vi "combine time and data into a single array.vi"() -> ()   [LabVIEW 2011]
uses:
  <vilib>/Utility/file.llb/Write To Spreadsheet File (DBL).vi
panel:
  in  "name of file":string="test data.txt"
  in  "export path 2":path=path "C:/Users/VGroup/Desktop/testing file"
  in  "seconds to wait":u32=1
  in  "stop":bool
  out "appended array":dbl[](array[numeric])=[51.0, 140621.0, 200625.0, 0.14448535757155878]
  out "date number":i32=140621
  out "time number":i32=200625
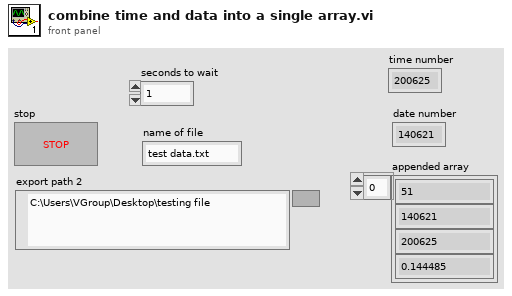
[diagram p1: front panel]
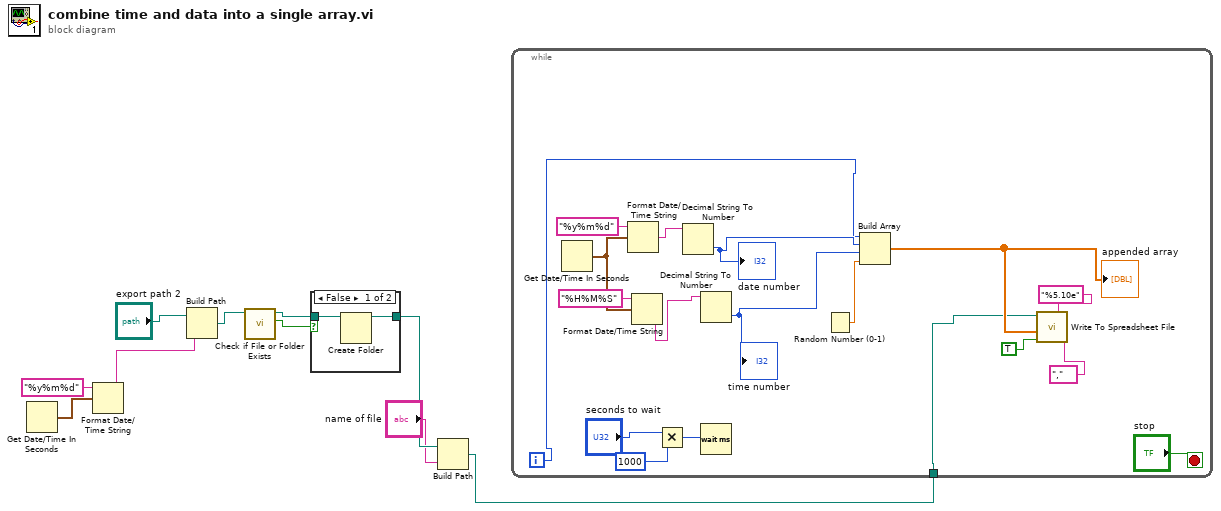
[diagram p0: block diagram]
diagram:
  n1 = Get Date/Time In Seconds() -> (seconds since 1Jan1904=w6:timestamp)
  n2 = Format Date/Time String(time format string (%c)="%y%m%d", seconds (now)=w6) -> (date/time string=w5:string)  [unwired: 1 in]
  n3 = Build Path(base path="export path 2", name or relative path=w5) -> (appended path=w3:path)
  n4 = call <vilib>:"Check if File or Folder Exists.vi"("path"=w3) -> ("file or folder exists?"=w1:bool, "dup path"=w2:path)  [unwired: 8 in, 1 out]
  n5 = case shown="False" w1 {
    tunnel: [w12 w13] -> w9
    tunnel: w2 -> [w11 w13]
    frame False {
      n6 = Create Folder(path (use dialog)=w11) -> (created path=w12:path)  [unwired: 2 in, 2 out]
    }
    frame True {
    }
  }
  n7 = Build Path(base path=w9, name or relative path="name of file") -> (appended path=w7:path)
  n8 = while {
    tunnel: w7 -> [w17]
    i -> [w21]
    stop <- "stop" stop-if-true
    n9 = Get Date/Time In Seconds() -> (seconds since 1Jan1904=w31:timestamp)
    n10 = Format Date/Time String(time format string (%c)="%y%m%d", seconds (now)=w31) -> (date/time string=w14:string)  [unwired: 1 in]
    n11 = Format Date/Time String(time format string (%c)="%H%M%S", seconds (now)=w31) -> (date/time string=w30:string)  [unwired: 1 in]
    n12 = Multiply(x="seconds to wait", y=u32 1000) -> (x*y=w18:u32)
    n13 = Decimal String To Number(string=w14) -> (number=w28:i32)  [unwired: 2 in, 1 out]
    "date number" <- w28
    n14 = Decimal String To Number(string=w30) -> (number=w27:i32)  [unwired: 2 in, 1 out]
    "time number" <- w27
    n15 = Wait (ms)(milliseconds to wait=w18) -> ()  [unwired: 1 out]
    n16 = Random Number (0-1)() -> (number: 0 to 1=w29:dbl)
    n17 = Build Array(w21, w28, w27, w29) -> (w24:dbl[])
    "appended array" <- w24
    n18 = call-poly <vilib>:"Write To Spreadsheet File.vi"("delimiter (\\t)"="," ("delimiter (Tab)"), "format (%.3f)"="%5.10e", "append to file? (new file:F)"=TRUE ("transpose? (no:F)"), "1D data"=w24, "file path (dialog if empty)"=w17) -> ()  [unwired: 3 in, 1 out]
  }
